vi "test_GetElements.vi"() -> ()   [LabVIEW 2013]
panel:
  in  "Enum":enum16{"ItemA", "Item B", "Item C#"}(ring)=enum."Item C#"
  out "enum elements":string[](array[string])
  out "cluster elements":string[](array[string])
  out "interleaved array":u8[](array[numeric]) format="%.0x"
  in  "Cluster":T1
  # "length\nxE = 14"
  # "#elements"
  # "length\nx6 = 6"
  # "length\nx6 = 7"
  # "length\nx5 = 5"
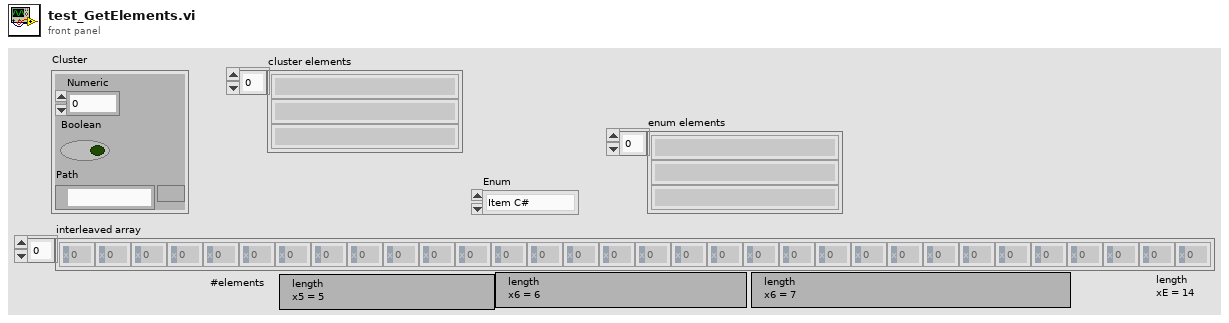
[diagram p1: front panel]
types:
  T1 = cluster{"Numeric":i32, "Boolean":bool, "Path":path}
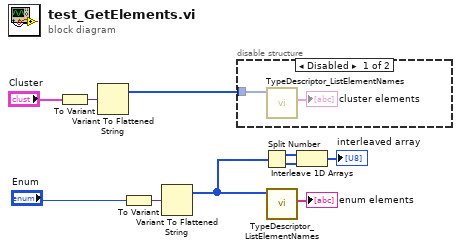
[diagram p0: block diagram]
diagram:
  n1 = To Variant(anything="Cluster") -> (Variant=w9:variant)
  n2 = Variant To Flattened String(Variant=w9) -> (1:w8:i16[])  [unwired: 1 out]
  n3 = To Variant(anything="Enum") -> (Variant=w4:variant)
  n4 = Variant To Flattened String(Variant=w4) -> (1:w1:i16[])  [unwired: 1 out]
  n5 = disable-structure shown="Disabled" {
    disable-tunnel: w8 -> [w12 _]
    frame Disabled {
      n6 = call "TypeDescriptor_ListElementNames.vi"("type descriptor"=w12) -> ("element names"=→"cluster elements":string[])  [unwired: 8 in, 2 out]
    }
    frame Enabled {
    }
  }
  n7 = Split Number(x=w1) -> (hi(x)=w7:u8[], lo(x)=w6:u8[])
  n8 = call "TypeDescriptor_ListElementNames.vi"("type descriptor"=w1) -> ("element names"=→"enum elements":string[])  [unwired: 8 in, 2 out]
  n9 = Interleave 1D Arrays(w7, w6) -> (→"interleaved array":u8[])
